vi "PWM_Count_1.vi"() -> ()   [LabVIEW 2019]
uses:
  <vilib>/rvi/Emulation/niFpgaGetClockAttributes.vi
  <vilib>/rvi/Emulation/niFpgaSctlEmulationGetInTimedLoop.vi
  <vilib>/rvi/Emulation/niFpgaEmulationReportErrorSimple.vi
  <vilib>/rvi/eio/common/nirviEmuTemplateMethod_errors.vi
  <vilib>/rvi/Emulation/niFpgaCriticalErrorInLSC.vi
  <vilib>/eio/EIONode/EIONode.xnode
panel:
  out "波形图表":u32(graph)
  out "x-y":u32
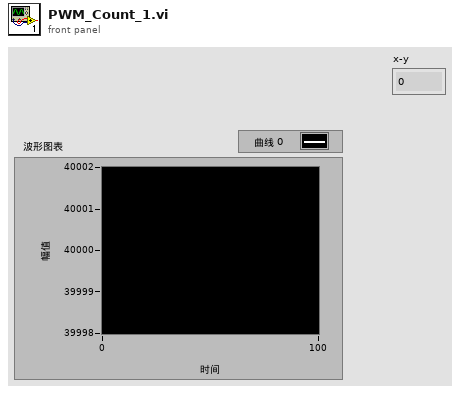
[diagram p1: front panel]
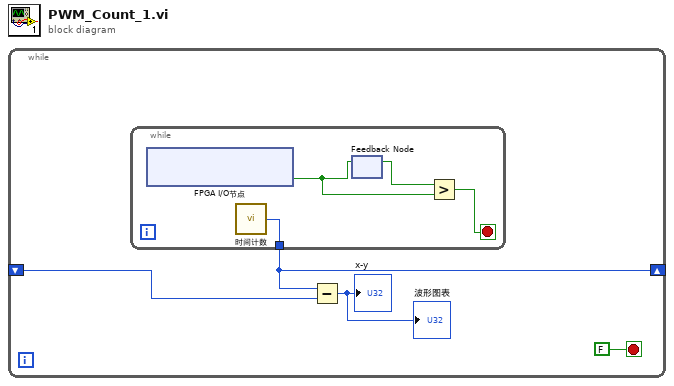
[diagram p0: block diagram]
diagram:
  n1 = while {
    shift-right: [w3] -> _
    shift-left: _ -> [w2]
    stop <- FALSE stop-if-true
    n2 = while {
      tunnel: [w5] -> w3
      stop <- w6 stop-if-true
      n3 = xnode "FPGA I/O节点"() -> ("ConnectorB/DIO0"=w7:bool)  [unwired: 1 in, 1 out]
      n4 = call "时间计数"() -> ("Tick Count(Ticks)"=w5:u32)
      n5 = feedback #1() -> (w8:bool)  [unwired: 1 in]
      n6 = feedback-in #1(w7) -> ()
      n7 = Greater?(x=w8, y=w7) -> (0:w6:bool)
    }
    n8 = Subtract(x=w3, y=w2) -> (x-y=→"x-y" →"波形图表":u32)
  }
